vi "GeoData.vi"() -> ()   [LabVIEW 2017] (continued)
H1\n27320\t37157\tReidsville\tNC\tRockingham County\tH1\n27375\t37157\tWentworth\tNC\tRockingham County\tH1\n27357\t37157\tStokesdale\tNC\tRockingham County\tH1\n27358\t37157\tSummerfield\tNC\tRockingham County\tH1\n27214\t37157\tBrowns summit\tNC\tRockingham County\tH1\n27288\t37157\tEden\tNC\tRockingham County\tH1\n27027\t37157\tMayodan\tNC\tRockingham County\tH1\n27025\t37157\tMadison\tNC\tRockingham County\tH1\n27249\t37157\tGibsonville\tNC\tRockingham County\tH1\n27289\t37157\tEden\tNC\tRockingham County\tH1\n27311\t37157\tPelham\tNC\tRockingham County\tH1\n28147\t37159\tSalisbury\tNC\tRowan County\tH1\n28159\t37159\tSpencer\tNC\tRowan County\tH1\n28039\t37159\tEast spencer\tNC\tRowan County\tH1\n28146\t37159\tSalisbury\tNC\tRowan County\tH1\n27054\t37159\tWoodleaf\tNC\tRowan County\tH1\n28023\t37159\tChina grove\tNC\tRowan County\tH1\n28127\t37159\tNew london\tNC\tRowan County\tH1\n28072\t37159\tGranite quarry\tNC\tRowan County\tH1\n28083\t37159\tKannapolis\tNC\tRowan County\tH1\n28137\t37159\tRichfield\tNC\tRowan County\tH1\n28071\t37159\tGold hill\tNC\tRowan County\tH1\n28088\t37159\tLandis\tNC\tRowan County\tH1\n28138\t37159\tRockwell\tNC\tRowan County\tH1\n28125\t37159\tMount ulla\tNC\tRowan County\tH1\n28145\t37159\tSalisbury\tNC\tRowan County\tH1\n28625\t37159\tStatesville\tNC\tRowan County\tH1\n28036\t37159\tDavidson\tNC\tRowan County\tH1\n28081\t37159\tKannapolis\tNC\tRowan County\tH1\n28144\t37159\tSalisbury\tNC\tRowan County\tH1\n28041\t37159\tFaith\tNC\tRowan County\tH1\n27013\t37159\tCleveland\tNC\tRowan County\tH1\n28115\t37159\tMooresville\tNC\tRowan County\tH1\n28167\t37161\tUnion mills\tNC\tRutherford County\tH1\n28752\t37161\tMarion\tNC\tRutherford County\tH1\n28024\t37161\tCliffside\tNC\tRutherford County\tH1\n28139\t37161\tRutherfordton\tNC\tRutherford County\tH1\n28756\t37161\tMill spring\tNC\tRutherford County\tH1\n28076\t37161\tHenrietta\tNC\tRutherford County\tH1\n28019\t37161\tCaroleen\tNC\tRutherford County\tH1\n28746\t37161\tLake lure\tNC\tRutherford County\tH1\n28018\t37161\tBostic\tNC\tRutherford County\tH1\n28043\t37161\tForest city\tNC\tRutherford County\tH1\n28150\t37161\tShelby\tNC\tRutherford County\tH1\n28020\t37161\tCasar\tNC\tRutherford County\tH1\n28711\t37161\tBlack mountain\tNC\tRutherford County\tH1\n28160\t37161\tSpindale\tNC\tRutherford County\tH1\n28074\t37161\tHarris\tNC\tRutherford County\tH1\n28040\t37161\tEllenboro\tNC\tRutherford County\tH1\n28114\t37161\tMooresboro\tNC\tRutherford County\tH1\n28720\t37161\tChimney rock\tNC\tRutherford County\tH1\n28334\t37163\tDunn\tNC\tSampson County\tH1\n28458\t37163\tRose hill\tNC\tSampson County\tH1\n28393\t37163\tTurkey\tNC\tSampson County\tH1\n28328\t37163\tClinton\tNC\tSampson County\tH1\n28365\t37163\tMount olive\tNC\tSampson County\tH1\n28444\t37163\tHarrells\tNC\tSampson County\tH1\n28329\t37163\tClinton\tNC\tSampson County\tH1\n28366\t37163\tNewton grove\tNC\tSampson County\tH1\n28385\t37163\tSalemburg\tNC\tSampson County\tH1\n28341\t37163\tFaison\tNC\tSampson County\tH1\n28344\t37163\tGodwin\tNC\tSampson County\tH1\n28453\t37163\tMagnolia\tNC\tSampson County\tH1\n28382\t37163\tRoseboro\tNC\tSampson County\tH1\n28391\t37163\tStedman\tNC\tSampson County\tH1\n28398\t37163\tWarsaw\tNC\tSampson County\tH1\n28447\t37163\tIvanhoe\tNC\tSampson County\tH1\n28318\t37163\tAutryville\tNC\tSampson County\tH1\n28478\t37163\tWillard\tNC\tSampson County\tH1\n28421\t37163\tAtkinson\tNC\tSampson County\tH1\n28441\t37163\tGarland\tNC\tSampson County\tH1\n28466\t37163\tWallace\tNC\tSampson County\tH1\n28352\t37165\tLaurinburg\tNC\tScotland County\tH1\n28364\t37165\tMaxton\tNC\tScotland County\tH1\n28396\t37165\tWagram\tNC\tScotland County\tH1\n28363\t37165\tMarston\tNC\tScotland County\tH1\n28351\t37165\tLaurel hill\tNC\tScotland County\tH1\n28343\t37165\tGibson\tNC\tScotland County\tH1\n28345\t37165\tHamlet\tNC\tScotland County\tH1\n28353\t37165\tLaurinburg\tNC\tScotland County\tH1\n28009\t37167\tBadin\tNC\tStanly County\tH1\n28002\t37167\tAlbemarle\tNC\tStanly County\tH1\n28127\t37167\tNew london\tNC\tStanly County\tH1\n28001\t37167\tAlbemarle\tNC\tStanly County\tH1\n28097\t37167\tLocust\tNC\tStanly County\tH1\n28129\t37167\tOakboro\tNC\tStanly County\tH1\n28163\t37167\tStanfield\tNC\tStanly County\tH1\n28137\t37167\tRichfield\tNC\tStanly County\tH1\n28109\t37167\tMisenheimer\tNC\tStanly County\tH1\n28071\t37167\tGold hill\tNC\tStanly County\tH1\n28107\t37167\tMidland\tNC\tStanly County\tH1\n28128\t37167\tNorwood\tNC\tStanly County\tH1\n28124\t37167\tMount pleasant\tNC\tStanly County\tH1\n27009\t37169\tBelews creek\tNC\tStokes County\tH1\n27046\t37169\tSandy ridge\tNC\tStokes County\tH1\n27021\t37169\tKing\tNC\tStokes County\tH1\n27043\t37169\tPinnacle\tNC\tStokes County\tH1\n27045\t37169\tRural hall\tNC\tStokes County\tH1\n27022\t37169\tLawsonville\tNC\tStokes County\tH1\n27042\t37169\tPine hall\tNC\tStokes County\tH1\n27041\t37169\tPilot mountain\tNC\tStokes County\tH1\n27019\t37169\tGermanton\tNC\tStokes County\tH1\n27053\t37169\tWestfield\tNC\tStokes County\tH1\n27052\t37169\tWalnut cove\tNC\tStokes County\tH1\n27357\t37169\tStokesdale\tNC\tStokes County\tH1\n27016\t37169\tDanbury\tNC\tStokes County\tH1\n27030\t37169\tMount airy\tNC\tStokes County\tH1\n27050\t37169\tTobaccoville\tNC\tStokes County\tH1\n27025\t37169\tMadison\tNC\tStokes County\tH1\n27043\t37171\tPinnacle\tNC\tSurry County\tH1\n27047\t37171\tSiloam\tNC\tSurry County\tH1\n28669\t37171\tRoaring river\tNC\tSurry County\tH1\n28676\t37171\tState road\tNC\tSurry County\tH1\n27024\t37171\tLowgap\tNC\tSurry County\tH1\n28621\t37171\tElkin\tNC\tSurry County\tH1\n27049\t37171\tToast\tNC\tSurry County\tH1\n27041\t37171\tPilot mountain\tNC\tSurry County\tH1\n27053\t37171\tWestfield\tNC\tSurry County\tH1\n28683\t37171\tThurmond\tNC\tSurry County\tH1\n27030\t37171\tMount airy\tNC\tSurry County\tH1\n27017\t37171\tDobson\tNC\tSurry County\tH1\n27007\t37171\tArarat\tNC\tSurry County\tH1\n28713\t37173\tBryson city\tNC\tSwain County\tH1\n28719\t37173\tCherokee\tNC\tSwain County\tH1\n28702\t37173\tAlmond\tNC\tSwain County\tH1\n28789\t37173\tWhittier\tNC\tSwain County\tH1\n28771\t37173\tRobbinsville\tNC\tSwain County\tH1\n28708\t37175\tBalsam grove\tNC\tTransylvania County\tH1\n28718\t37175\tCedar mountain\tNC\tTransylvania County\tH1\n28747\t37175\tLake toxaway\tNC\tTransylvania County\tH1\n28766\t37175\tPenrose\tNC\tTransylvania County\tH1\n28739\t37175\tHendersonville\tNC\tTransylvania County\tH1\n28742\t37175\tHorse shoe\tNC\tTransylvania County\tH1\n28712\t37175\tBrevard\tNC\tTransylvania County\tH1\n28768\t37175\tPisgah forest\tNC\tTransylvania County\tH1\n28772\t37175\tRosman\tNC\tTransylvania County\tH1\n28783\t37175\tTuckasegee\tNC\tTransylvania County\tH1\n28774\t37175\tSapphire\tNC\tTransylvania County\tH1\n28759\t37175\tMills river\tNC\tTransylvania County\tH1\n27826\t37177\tFairfield\tNC\tTyrrell County\tH1\n27925\t37177\tColumbia\tNC\tTyrrell County\tH1\n27928\t37177\tCreswell\tNC\tTyrrell County\tH1\n28108\t37179\tMineral springs\tNC\tUnion County\tH1\n28135\t37179\tPolkton\tNC\tUnion County\tH1\n28133\t37179\tPeachland\tNC\tUnion County\tH1\n28227\t37179\tCharlotte\tNC\tUnion County\tH1\n28103\t37179\tMarshville\tNC\tUnion County\tH1\n28105\t37179\tMatthews\tNC\tUnion County\tH1\n28112\t37179\tMonroe\tNC\tUnion County\tH1\n28107\t37179\tMidland\tNC\tUnion County\tH1\n28111\t37179\tMonroe\tNC\tUnion County\tH1\n28174\t37179\tWingate\tNC\tUnion County\tH1\n28079\t37179\tIndian trail\tNC\tUnion County\tH1\n28173\t37179\tWaxhaw\tNC\tUnion County\tH1\n28104\t37179\tMatthews\tNC\tUnion County\tH1\n28110\t37179\tMonroe\tNC\tUnion County\tH1\n27537\t37181\tHenderson\tNC\tVance County\tH1\n27553\t37181\tManson\tNC\tVance County\tH1\n27565\t37181\tOxford\tNC\tVance County\tH1\n27556\t37181\tMiddleburg\tNC\tVance County\tH1\n27507\t37181\tBullock\tNC\tVance County\tH1\n27536\t37181\tHenderson\tNC\tVance County\tH1\n27563\t37181\tNorlina\tNC\tVance County\tH1\n27544\t37181\tKittrell\tNC\tVance County\tH1\n27584\t37181\tTownsville\tNC\tVance County\tH1\n27512\t37183\tCary\tNC\tWake County\tH1\n27587\t37183\tWake forest\tNC\tWake County\tH1\n27610\t37183\tRaleigh\tNC\tWake County\tH1\n27614\t37183\tRaleigh\tNC\tWake County\tH1\n27640\t37183\tRaleigh\tNC\tWake County\tH1\n27502\t37183\tApex\tNC\tWake County\tH1\n27519\t37183\tCary\tNC\tWake County\tH1\n27526\t37183\tFuquay varina\tNC\tWake County\tH1\n27562\t37183\tNew hill\tNC\tWake County\tH1\n27619\t37183\tRaleigh\tNC\tWake County\tH1\n27699\t37183\tRaleigh\tNC\tWake County\tH1\n27690\t37183\tRaleigh\tNC\tWake County\tH1\n27661\t37183\tRaleigh\tNC\tWake County\tH1\n27501\t37183\tAngier\tNC\tWake County\tH1\n27604\t37183\tRaleigh\tNC\tWake County\tH1\n27596\t37183\tYoungsville\tNC\tWake County\tH1\n27713\t37183\tDurham\tNC\tWake County\tH1\n27628\t37183\tRaleigh\tNC\tWake County\tH1\n27520\t37183\tClayton\tNC\tWake County\tH1\n27518\t37183\tCary\tNC\tWake County\tH1\n27545\t37183\tKnightdale\tNC\tWake County\tH1\n27560\t37183\tMorrisville\tNC\tWake County\tH1\n27592\t37183\tWillow spring\tNC\tWake County\tH1\n27609\t37183\tRaleigh\tNC\tWake County\tH1\n27615\t37183\tRaleigh\tNC\tWake County\tH1\n27622\t37183\tRaleigh\tNC\tWake County\tH1\n27629\t37183\tRaleigh\tNC\tWake County\tH1\n27675\t37183\tRaleigh\tNC\tWake County\tH1\n27611\t37183\tRaleigh\tNC\tWake County\tH1\n27513\t37183\tCary\tNC\tWake County\tH1\n27522\t37183\tCreedmoor\tNC\tWake County\tH1\n27529\t37183\tGarner\tNC\tWake County\tH1\n27656\t37183\tRaleigh\tNC\tWake County\tH1\n27511\t37183\tCary\tNC\tWake County\tH1\n27523\t37183\tApex\tNC\tWake County\tH1\n27591\t37183\tWendell\tNC\tWake County\tH1\n27603\t37183\tRaleigh\tNC\tWake County\tH1\n27605\t37183\tRaleigh\tNC\tWake County\tH1\n27607\t37183\tRaleigh\tNC\tWake County\tH1\n27608\t37183\tRaleigh\tNC\tWake County\tH1\n27613\t37183\tRaleigh\tNC\tWake County\tH1\n27616\t37183\tRaleigh\tNC\tWake County\tH1\n27588\t37183\tWake forest\tNC\tWake County\tH1\n27636\t37183\tRaleigh\tNC\tWake County\tH1\n27697\t37183\tRaleigh\tNC\tWake County\tH1\n27602\t37183\tRaleigh\tNC\tWake County\tH1\n27601\t37183\tRaleigh\tNC\tWake County\tH1\n27606\t37183\tRaleigh\tNC\tWake County\tH1\n27612\t37183\tRaleigh\tNC\tWake County\tH1\n27617\t37183\tRaleigh\tNC\tWake County\tH1\n27703\t37183\tDurham\tNC\tWake County\tH1\n27571\t37183\tRolesville\tNC\tWake County\tH1\n27620\t37183\tRaleigh\tNC\tWake County\tH1\n27623\t37183\tRaleigh\tNC\tWake County\tH1\n27540\t37183\tHolly springs\tNC\tWake County\tH1\n27539\t37183\tApex\tNC\tWake County\tH1\n27597\t37183\tZebulon\tNC\tWake County\tH1\n27627\t37183\tRaleigh\tNC\tWake County\tH1\n27624\t37183\tRaleigh\tNC\tWake County\tH1\n27658\t37183\tRaleigh\tNC\tWake County\tH1\n27676\t37183\tRaleigh\tNC\tWake County\tH1\n27537\t37185\tHenderson\tNC\tWarren County\tH1\n27551\t37185\tMacon\tNC\tWarren County\tH1\n27553\t37185\tManson\tNC\tWarren County\tH1\n27850\t37185\tLittleton\tNC\tWarren County\tH1\n27589\t37185\tWarrenton\tNC\tWarren County\tH1\n27844\t37185\tHollister\tNC\tWarren County\tH1\n27586\t37185\tVaughan\tNC\tWarren County\tH1\n27563\t37185\tNorlina\tNC\tWarren County\tH1\n27594\t37185\tWise\tNC\tWarren County\tH1\n27570\t37185\tRidgeway\tNC\tWarren County\tH1\n27842\t37185\tHenrico\tNC\tWarren County\tH1\n27860\t37187\tPantego\tNC\tWashington County\tH1\n27962\t37187\tPlymouth\tNC\tWashington County\tH1\n27970\t37187\tRoper\tNC\tWashington County\tH1\n27928\t37187\tCreswell\tNC\tWashington County\tH1\n27865\t37187\tPinetown\tNC\tWashington County\tH1\n28622\t37189\tElk park\tNC\tWatauga County\tH1\n28604\t37189\tBanner elk\tNC\tWatauga County\tH1\n28645\t37189\tLenoir\tNC\tWatauga County\tH1\n28608\t37189\tBoone\tNC\tWatauga County\tH1\n28698\t37189\tZionville\tNC\tWatauga County\tH1\n28607\t37189\tBoone\tNC\tWatauga County\tH1\n28605\t37189\tBlowing rock\tNC\tWatauga County\tH1\n28692\t37189\tVilas\tNC\tWatauga County\tH1\n28618\t37189\tDeep gap\tNC\tWatauga County\tH1\n28684\t37189\tTodd\tNC\tWatauga County\tH1\n28679\t37189\tSugar grove\tNC\tWatauga County\tH1\n27542\t37191\tKenly\tNC\tWayne County\tH1\n27524\t37191\tFour oaks\tNC\tWayne County\tH1\n27863\t37191\tPikeville\tNC\tWayne County\tH1\n28333\t37191\tDudley\tNC\tWayne County\tH1\n28365\t37191\tMount olive\tNC\tWayne County\tH1\n27533\t37191\tGoldsboro\tNC\tWayne County\tH1\n27569\t37191\tPrinceton\tNC\tWayne County\tH1\n27531\t37191\tGoldsboro\tNC\tWayne County\tH1\n27830\t37191\tFremont\tNC\tWayne County\tH1\n28578\t37191\tSeven springs\tNC\tWayne County\tH1\n27532\t37191\tGoldsboro\tNC\tWayne County\tH1\n27534\t37191\tGoldsboro\tNC\tWayne County\tH1\n27851\t37191\tLucama\tNC\tWayne County\tH1\n27530\t37191\tGoldsboro\tNC\tWayne County\tH1\n27883\t37191\tStantonsburg\tNC\tWayne County\tH1\n28551\t37191\tLa grange\tNC\tWayne County\tH1\n28635\t37193\tHays\tNC\tWilkes County\tH1\n28651\t37193\tMillers creek\tNC\tWilkes County\tH1\n28670\t37193\tRonda\tNC\tWilkes County\tH1\n28624\t37193\tFerguson\tNC\tWilkes County\tH1\n28645\t37193\tLenoir\tNC\tWilkes County\tH1\n28644\t37193\tLaurel springs\tNC\tWilkes County\tH1\n28669\t37193\tRoaring river\tNC\tWilkes County\tH1\n28676\t37193\tState road\tNC\tWilkes County\tH1\n28621\t37193\tElkin\tNC\tWilkes County\tH1\n28659\t37193\tNorth wilkesboro\tNC\tWilkes County\tH1\n28654\t37193\tMoravian falls\tNC\tWilkes County\tH1\n28642\t37193\tJonesville\tNC\tWilkes County\tH1\n28685\t37193\tTraphill\tNC\tWilkes County\tH1\n28683\t37193\tThurmond\tNC\tWilkes County\tH1\n28618\t37193\tDeep gap\tNC\tWilkes County\tH1\n28665\t37193\tPurlear\tNC\tWilkes County\tH1\n28649\t37193\tMc grady\tNC\tWilkes County\tH1\n28606\t37193\tBoomer\tNC\tWilkes County\tH1\n28694\t37193\tWest jefferson\tNC\tWilkes County\tH1\n27020\t37193\tHamptonville\tNC\tWilkes County\tH1\n28697\t37193\tWilkesboro\tNC\tWilkes County\tH1\n28689\t37193\tUnion grove\tNC\tWilkes County\tH1\n28656\t37193\tNorth wilkesboro\tNC\tWilkes County\tH1\n27542\t37195\tKenly\tNC\tWilson County\tH1\n27894\t37195\tWilson\tNC\tWilson County\tH1\n27803\t37195\tRocky mount\tNC\tWilson County\tH1\n27807\t37195\tBailey\tNC\tWilson County\tH1\n27852\t37195\tMacclesfield\tNC\tWilson County\tH1\n27822\t37195\tElm city\tNC\tWilson County\tH1\n27880\t37195\tSims\tNC\tWilson County\tH1\n27893\t37195\tWilson\tNC\tWilson County\tH1\n27829\t37195\tFountain\tNC\tWilson County\tH1\n27888\t37195\tWalstonburg\tNC\tWilson County\tH1\n27830\t37195\tFremont\tNC\tWilson County\tH1\n27895\t37195\tWilson\tNC\tWilson County\tH1\n27873\t37195\tSaratoga\tNC\tWilson County\tH1\n27896\t37195\tWilson\tNC\tWilson County\tH1\n27813\t37195\tBlack creek\tNC\tWilson County\tH1\n27851\t37195\tLucama\tNC\tWilson County\tH1\n27557\t37195\tMiddlesex\tNC\tWilson County\tH1\n27883\t37195\tStantonsburg\tNC\tWilson County\tH1\n27011\t37197\tBoonville\tNC\tYadkin County\tH1\n28634\t37197\tHarmony\tNC\tYadkin County\tH1\n27018\t37197\tEast bend\tNC\tYadkin County\tH1\n28642\t37197\tJonesville\tNC\tYadkin County\tH1\n27020\t37197\tHamptonville\tNC\tYadkin County\tH1\n27055\t37197\tYadkinville\tNC\tYadkin County\tH1\n28689\t37197\tUnion grove\tNC\tYadkin County\tH1\n28714\t37199\tBurnsville\tNC\tYancey County\tH1\n28777\t37199\tSpruce pine\tNC\tYancey County\tH1\n28755\t37199\tMicaville\tNC\tYancey County\tH1\n28740\t37199\tGreen mountain\tNC\tYancey County\tH1\n28754\t37199\tMars hill\tNC\tYancey County\tH1\n28705\t37199\tBakersville\tNC\tYancey County\tH1\n58639\t38001\tHettinger\tND\tAdams County\tH1\n58562\t38001\tNew leipzig\tND\tAdams County\tH1\n58649\t38001\tReeder\tND\tAdams County\tH1\n58646\t38001\tMott\tND\tAdams County\tH1\n58650\t38001\tRegent\tND\tAdams County\tH1\n58479\t38003\tRogers\tND\tBarnes County\tH1\n58492\t38003\tWimbledon\tND\tBarnes County\tH1\n58466\t38003\tMarion\tND\tBarnes County\tH1\n58065\t38003\tPillsbury\tND\tBarnes County\tH1\n58072\t38003\tValley city\tND\tBarnes County\tH1\n58062\t38003\tNome\tND\tBarnes County\tH1\n58481\t38003\tSpiritwood\tND\tBarnes County\tH1\n58031\t38003\tFingal\tND\tBarnes County\tH1\n58056\t38003\tLuverne\tND\tBarnes County\tH1\n58497\t38003\tYpsilanti\tND\tBarnes County\tH1\n58064\t38003\tPage\tND\tBarnes County\tH1\n58049\t38003\tKathryn\tND\tBarnes County\tH1\n58027\t38003\tEnderlin\tND\tBarnes County\tH1\n58071\t38003\tTower city\tND\tBarnes County\tH1\n58063\t38003\tOriska\tND\tBarnes County\tH1\n58461\t38003\tLitchville\tND\tBarnes County\tH1\n58480\t38003\tSanborn\tND\tBarnes County\tH1\n58046\t38003\tHope\tND\tBarnes County\tH1\n58429\t38003\tDazey\tND\tBarnes County\tH1\n58374\t38005\tSheyenne\tND\tBenson County\tH1\n58348\t38005\tMaddock\tND\tBenson County\tH1\n58381\t38005\tWarwick\tND\tBenson County\tH1\n58357\t38005\tOberon\tND\tBenson County\tH1\n58335\t38005\tFort totten\tND\tBenson County\tH1\n58301\t38005\tDevils lake\tND\tBenson County\tH1\n58332\t38005\tEsmond\tND\tBenson County\tH1\n58370\t38005\tSaint michael\tND\tBenson County\tH1\n58368\t38005\tRugby\tND\tBenson County\tH1\n58386\t38005\tYork\tND\tBenson County\tH1\n58343\t38005\tKnox\tND\tBenson County\tH1\n58325\t38005\tChurchs ferry\tND\tBenson County\tH1\n58380\t38005\tTolna\tND\tBenson County\tH1\n58341\t38005\tHarvey\tND\tBenson County\tH1\n58385\t38005\tWolford\tND\tBenson County\tH1\n58346\t38005\tLeeds\tND\tBenson County\tH1\n58351\t38005\tMinnewaukan\tND\tBenson County\tH1\n58379\t38005\tTokio\tND\tBenson County\tH1\n58622\t38007\tBelfield\tND\tBillings County\tH1\n58620\t38007\tAmidon\tND\tBillings County\tH1\n58645\t38007\tMedora\tND\tBillings County\tH1\n58640\t38007\tKilldeer\tND\tBillings County\tH1\n58627\t38007\tFairfield\tND\tBillings County\tH1\n58634\t38007\tGrassy butte\tND\tBillings County\tH1\n58642\t38007\tManning\tND\tBillings County\tH1\n58750\t38009\tLansford\tND\tBottineau County\tH1\n58740\t38009\tGlenburn\tND\tBottineau County\tH1\n58711\t38009\tAntler\tND\tBottineau County\tH1\n58762\t38009\tNewburg\tND\tBottineau County\tH1\n58384\t38009\tWillow city\tND\tBottineau County\tH1\n58760\t38009\tMaxbass\tND\tBottineau County\tH1\n58318\t38009\tBottineau\tND\tBottineau County\tH1\n58782\t38009\tSherwood\tND\tBottineau County\tH1\n58783\t38009\tSouris\tND\tBottineau County\tH1\n58789\t38009\tUpham\tND\tBottineau County\tH1\n58793\t38009\tWesthope\tND\tBottineau County\tH1\n58329\t38009\tDunseith\tND\tBottineau County\tH1\n58761\t38009\tMohall\tND\tBottineau County\tH1\n58748\t38009\tKramer\tND\tBottineau County\tH1\n58643\t38011\tMarmarth\tND\tBowman County\tH1\n58651\t38011\tRhame\tND\tBowman County\tH1\n58653\t38011\tScranton\tND\tBowman County\tH1\n58623\t38011\tBowman\tND\tBowman County\tH1\n58649\t38011\tReeder\tND\tBowman County\tH1\n58737\t38013\tFlaxton\tND\tBurke County\tH1\n58784\t38013\tStanley\tND\tBurke County\tH1\n58727\t38013\tColumbus\tND\tBurke County\tH1\n58772\t38013\tPortal\tND\tBurke County\tH1\n58755\t38013\tMcgregor\tND\tBurke County\tH1\n58721\t38013\tBowbells\tND\tBurke County\tH1\n58773\t38013\tPowers lake\tND\tBurke County\tH1\n58752\t38013\tLignite\tND\tBurke County\tH1\n58746\t38013\tKenmare\tND\tBurke County\tH1\n58504\t38015\tBismarck\tND\tBurleigh County\tH1\n58521\t38015\tBaldwin\tND\tBurleigh County\tH1\n58505\t38015\tBismarck\tND\tBurleigh County\tH1\n58501\t38015\tBismarck\tND\tBurleigh County\tH1\n58524\t38015\tBraddock\tND\tBurleigh County\tH1\n58572\t38015\tSterling\tND\tBurleigh County\tH1\n58579\t38015\tWilton\tND\tBurleigh County\tH1\n58502\t38015\tBismarck\tND\tBurleigh County\tH1\n58494\t38015\tWing\tND\tBurleigh County\tH1\n58532\t38015\tDriscoll\tND\tBurleigh County\tH1\n58477\t38015\tRegan\tND\tBurleigh County\tH1\n58560\t38015\tMoffit\tND\tBurleigh County\tH1\n58503\t38015\tBismarck\tND\tBurleigh County\tH1\n58506\t38015\tBismarck\tND\tBurleigh County\tH1\n58558\t38015\tMenoken\tND\tBurleigh County\tH1\n58507\t38015\tBismarck\tND\tBurleigh County\tH1\n58103\t38017\tFargo\tND\tCass County\tH1\n58006\t38017\tArthur\tND\tCass County\tH1\n58038\t38017\tGrandin\tND\tCass County\tH1\n58042\t38017\tHarwood\tND\tCass County\tH1\n58126\t38017\tFargo\tND\tCass County\tH1\n58047\t38017\tHorace\tND\tCass County\tH1\n58012\t38017\tCasselton\tND\tCass County\tH1\n58015\t38017\tChristine\tND\tCass County\tH1\n58104\t38017\tFargo\tND\tCass County\tH1\n58035\t38017\tGalesburg\tND\tCass County\tH1\n58105\t38017\tFargo\tND\tCass County\tH1\n58079\t38017\tWheatland\tND\tCass County\tH1\n58106\t38017\tFargo\tND\tCass County\tH1\n58002\t38017\tAbsaraka\tND\tCass County\tH1\n58031\t38017\tFingal\tND\tCass County\tH1\n58064\t38017\tPage\tND\tCass County\tH1\n58108\t38017\tFargo\tND\tCass County\tH1\n58125\t38017\tFargo\tND\tCass County\tH1\n58124\t38017\tFargo\tND\tCass County\tH1\n58027\t38017\tEnderlin\tND\tCass County\tH1\n58107\t38017\tFargo\tND\tCass County\tH1\n58048\t38017\tHunter\tND\tCass County\tH1\n58021\t38017\tDavenport\tND\tCass County\tH1\n58071\t38017\tTower city\tND\tCass County\tH1\n58004\t38017\tAmenia\tND\tCass County\tH1\n58109\t38017\tFargo\tND\tCass County\tH1\n58121\t38017\tFargo\tND\tCass County\tH1\n58078\t38017\tWest fargo\tND\tCass County\tH1\n58052\t38017\tLeonard\tND\tCass County\tH1\n58011\t38017\tBuffalo\tND\tCass County\tH1\n58029\t38017\tErie\tND\tCass County\tH1\n58051\t38017\tKindred\tND\tCass County\tH1\n58046\t38017\tHope\tND\tCass County\tH1\n58007\t38017\tAyr\tND\tCass County\tH1\n58036\t38017\tGardner\tND\tCass County\tH1\n58122\t38017\tFargo\tND\tCass County\tH1\n58102\t38017\tFargo\tND\tCass County\tH1\n58059\t38017\tMapleton\tND\tCass County\tH1\n58005\t38017\tArgusville\tND\tCass County\tH1\n58239\t38019\tHannah\tND\tCavalier County\tH1\n58330\t38019\tEdmore\tND\tCavalier County\tH1\n58338\t38019\tHampden\tND\tCavalier County\tH1\n58282\t38019\tWalhalla\tND\tCavalier County\tH1\n58377\t38019\tStarkweather\tND\tCavalier County\tH1\n58227\t38019\tEdinburg\tND\tCavalier County\tH1\n58352\t38019\tMunich\tND\tCavalier County\tH1\n58281\t38019\tWales\tND\tCavalier County\tH1\n58255\t38019\tMaida\tND\tCavalier County\tH1\n58269\t38019\tOsnabrock\tND\tCavalier County\tH1\n58260\t38019\tMilton\tND\tCavalier County\tH1\n58249\t38019\tLangdon\tND\tCavalier County\tH1\n58229\t38019\tFairdale\tND\tCavalier County\tH1\n58372\t38019\tSarles\tND\tCavalier County\tH1\n58311\t38019\tAlsen\tND\tCavalier County\tH1\n58262\t38019\tMountain\tND\tCavalier County\tH1\n58355\t38019\tNekoma\tND\tCavalier County\tH1\n58323\t38019\tCalvin\tND\tCavalier County\tH1\n58040\t38021\tGwinner\tND\tDickey County\tH1\n58439\t38021\tForbes\tND\tDickey County\tH1\n58456\t38021\tKulm\tND\tDickey County\tH1\n58436\t38021\tEllendale\tND\tDickey County\tH1\n58474\t38021\tOakes\tND\tDickey County\tH1\n58458\t38021\tLamoure\tND\tDickey County\tH1\n58441\t38021\tFullerton\tND\tDickey County\tH1\n58413\t38021\tAshley\tND\tDickey County\tH1\n58433\t38021\tEdgeley\tND\tDickey County\tH1\n58415\t38021\tBerlin\tND\tDickey County\tH1\n58845\t38023\tGrenora\tND\tDivide County\tH1\n58833\t38023\tAmbrose\tND\tDivide County\tH1\n58856\t38023\tZahl\tND\tDivide County\tH1\n58765\t38023\tNoonan\tND\tDivide County\tH1\n58755\t38023\tMcgregor\tND\tDivide County\tH1\n58830\t38023\tAlamo\tND\tDivide County\tH1\n58795\t38023\tWildrose\tND\tDivide County\tH1\n58730\t38023\tCrosby\tND\tDivide County\tH1\n58844\t38023\tFortuna\tND\tDivide County\tH1\n58601\t38025\tDickinson\tND\tDunn County\tH1\n58638\t38025\tHebron\tND\tDunn County\tH1\n58625\t38025\tDodge\tND\tDunn County\tH1\n58757\t38025\tMandaree\tND\tDunn County\tH1\n58636\t38025\tHalliday\tND\tDunn County\tH1\n58656\t38025\tTaylor\tND\tDunn County\tH1\n58626\t38025\tDunn center\tND\tDunn County\tH1\n58622\t38025\tBelfield\tND\tDunn County\tH1\n58644\t38025\tMarshall\tND\tDunn County\tH1\n58652\t38025\tRichardton\tND\tDunn County\tH1\n58640\t38025\tKilldeer\tND\tDunn County\tH1\n58854\t38025\tWatford city\tND\tDunn County\tH1\n58630\t38025\tGladstone\tND\tDunn County\tH1\n58642\t38025\tManning\tND\tDunn County\tH1\n58374\t38027\tSheyenne\tND\tEddy County\tH1\n58421\t38027\tCarrington\tND\tEddy County\tH1\n58381\t38027\tWarwick\tND\tEddy County\tH1\n58356\t38027\tNew rockford\tND\tEddy County\tH1\n58445\t38027\tGrace city\tND\tEddy County\tH1\n58380\t38027\tTolna\tND\tEddy County\tH1\n58464\t38027\tMchenry\tND\tEddy County\tH1\n58504\t38029\tBismarck\tND\tEmmons County\tH1\n58552\t38029\tLinton\tND\tEmmons County\tH1\n58524\t38029\tBraddock\tND\tEmmons County\tH1\n58544\t38029\tHazelton\tND\tEmmons County\tH1\n58549\t38029\tKintyre\tND\tEmmons County\tH1\n58581\t38029\tZeeland\tND\tEmmons County\tH1\n58495\t38029\tWishek\tND\tEmmons County\tH1\n58542\t38029\tHague\tND\tEmmons County\tH1\n58560\t38029\tMoffit\tND\tEmmons County\tH1\n58573\t38029\tStrasburg\tND\tEmmons County\tH1\n58443\t38031\tGlenfield\tND\tFoster County\tH1\n58421\t38031\tCarrington\tND\tFoster County\tH1\n58356\t38031\tNew rockford\tND\tFoster County\tH1\n58484\t38031\tSutton\tND\tFoster County\tH1\n58445\t38031\tGrace city\tND\tFoster County\tH1\n58464\t38031\tMchenry\tND\tFoster County\tH1\n58455\t38031\tKensal\tND\tFoster County\tH1\n58632\t38033\tGolva\tND\tGolden Valley County\tH1\n58645\t38033\tMedora\tND\tGolden Valley County\tH1\n58654\t38033\tSentinel butte\tND\tGolden Valley County\tH1\n58621\t38033\tBeach\tND\tGolden Valley County\tH1\n58261\t38035\tMinto\tND\tGrand Forks County\tH1\n58212\t38035\tAneta\tND\tGrand Forks County\tH1\n58228\t38035\tEmerado\tND\tGrand Forks County\tH1\n58278\t38035\tThompson\tND\tGrand Forks County\tH1\n58207\t38035\tGrand forks\tND\tGrand Forks County\tH1\n58256\t38035\tManvel\tND\tGrand Forks County\tH1\n58258\t38035\tMekinock\tND\tGrand Forks County\tH1\n58206\t38035\tGrand forks\tND\tGrand Forks County\tH1\n58203\t38035\tGrand forks\tND\tGrand Forks County\tH1\n58202\t38035\tGrand forks\tND\tGrand Forks County\tH1\n58231\t38035\tFordville\tND\tGrand Forks County\tH1\n58275\t38035\tReynolds\tND\tGrand Forks County\tH1\n58267\t38035\tNorthwood\tND\tGrand Forks County\tH1\n58205\t38035\tGrand forks afb\tND\tGrand Forks County\tH1\n58240\t38035\tHatton\tND\tGrand Forks County\tH1\n58266\t38035\tNiagara\tND\tGrand Forks County\tH1\n58201\t38035\tGrand forks\tND\tGrand Forks County\tH1\n58251\t38035\tLarimore\tND\tGrand Forks County\tH1\n58214\t38035\tArvilla\tND\tGrand Forks County\tH1\n58244\t38035\tInkster\tND\tGrand Forks County\tH1\n58204\t38035\tGrand forks afb\tND\tGrand Forks County\tH1\n58233\t38035\tForest river\tND\tGrand Forks County\tH1\n58208\t38035\tGrand forks\tND\tGrand Forks County\tH1\n58235\t38035\tGilby\tND\tGrand Forks County\tH1\n58638\t38037\tHebron\tND\tGrant County\tH1\n58569\t38037\tShields\tND\tGrant County\tH1\n58535\t38037\tFlasher\tND\tGrant County\tH1\n58520\t38037\tAlmont\tND\tGrant County\tH1\n58563\t38037\tNew salem\tND\tGrant County\tH1\n58562\t38037\tNew leipzig\tND\tGrant County\tH1\n58564\t38037\tRaleigh\tND\tGrant County\tH1\n58529\t38037\tCarson\tND\tGrant County\tH1\n58631\t38037\tGlen ullin\tND\tGrant County\tH1\n58533\t38037\tElgin\tND\tGrant County\tH1\n58212\t38039\tAneta\tND\tGriggs County\tH1\n58492\t38039\tWimbledon\tND\tGriggs County\tH1\n58416\t38039\tBinford\tND\tGriggs County\tH1\n58484\t38039\tSutton\tND\tGriggs County\tH1\n58056\t38039\tLuverne\tND\tGriggs County\tH1\n58448\t38039\tHannaford\tND\tGriggs County\tH1\n58464\t38039\tMchenry\tND\tGriggs County\tH1\n58425\t38039\tCooperstown\tND\tGriggs County\tH1\n58429\t38039\tDazey\tND\tGriggs County\tH1\n58452\t38039\tJessie\tND\tGriggs County\tH1\n58647\t38041\tNew england\tND\tHettinger County\tH1\n58562\t38041\tNew leipzig\tND\tHettinger County\tH1\n58646\t38041\tMott\tND\tHettinger County\tH1\n58650\t38041\tRegent\tND\tHettinger County\tH1\n58488\t38043\tTuttle\tND\tKidder County\tH1\n58524\t38043\tBraddock\tND\tKidder County\tH1\n58467\t38043\tMedina\tND\tKidder County\tH1\n58428\t38043\tDawson\tND\tKidder County\tH1\n58482\t38043\tSteele\tND\tKidder County\tH1\n58418\t38043\tBowdon\tND\tKidder County\tH1\n58549\t38043\tKintyre\tND\tKidder County\tH1\n58423\t38043\tChaseley\tND\tKidder County\tH1\n58483\t38043\tStreeter\tND\tKidder County\tH1\n58475\t38043\tPettibone\tND\tKidder County\tH1\n58532\t38043\tDriscoll\tND\tKidder County\tH1\n58496\t38043\tWoodworth\tND\tKidder County\tH1\n58478\t38043\tRobinson\tND\tKidder County\tH1\n58487\t38043\tTappen\tND\tKidder County\tH1\n58561\t38043\tNapoleon\tND\tKidder County\tH1\n58472\t38045\tMontpelier\tND\tLaMoure County\tH1\n58456\t38045\tKulm\tND\tLaMoure County\tH1\n58474\t38045\tOakes\tND\tLaMoure County\tH1\n58458\t38045\tLamoure\tND\tLaMoure County\tH1\n58466\t38045\tMarion\tND\tLaMoure County\tH1\n58490\t38045\tVerona\tND\tLaMoure County\tH1\n58033\t38045\tFort ransom\tND\tLaMoure County\tH1\n58431\t38045\tDickey\tND\tLaMoure County\tH1\n58049\t38045\tKathryn\tND\tLaMoure County\tH1\n58433\t38045\tEdgeley\tND\tLaMoure County\tH1\n58454\t38045\tJud\tND\tLaMoure County\tH1\n58461\t38045\tLitchville\tND\tLaMoure County\tH1\n58415\t38045\tBerlin\tND\tLaMoure County\tH1\n58442\t38045\tGackle\tND\tLaMoure County\tH1\n58440\t38047\tFredonia\tND\tLogan County\tH1\n58549\t38047\tKintyre\tND\tLogan County\tH1\n58483\t38047\tStreeter\tND\tLogan County\tH1\n58454\t38047\tJud\tND\tLogan County\tH1\n58460\t38047\tLehr\tND\tLogan County\tH1\n58495\t38047\tWishek\tND\tLogan County\tH1\n58561\t38047\tNapoleon\tND\tLogan County\tH1\n58442\t38047\tGackle\tND\tLogan County\tH1\n58768\t38049\tNorwich\tND\tMcHenry County\tH1\n58731\t38049\tDeering\tND\tMcHenry County\tH1\n58713\t38049\tBantry\tND\tMcHenry County\tH1\n58736\t38049\tDrake\tND\tMcHenry County\tH1\n58740\t38049\tGlenburn\tND\tMcHenry County\tH1\n58792\t38049\tVoltaire\tND\tMcHenry County\tH1\n58762\t38049\tNewburg\tND\tMcHenry County\tH1\n58384\t38049\tWillow city\tND\tMcHenry County\tH1\n58723\t38049\tButte\tND\tMcHenry County\tH1\n58741\t38049\tGranville\tND\tMcHenry County\tH1\n58712\t38049\tBalfour\tND\tMcHenry County\tH1\n58368\t38049\tRugby\tND\tMcHenry County\tH1\n58789\t38049\tUpham\tND\tMcHenry County\tH1\n58790\t38049\tVelva\tND\tMcHenry County\tH1\n58710\t38049\tAnamoose\tND\tMcHenry County\tH1\n58758\t38049\tMartin\tND\tMcHenry County\tH1\n58788\t38049\tTowner\tND\tMcHenry County\tH1\n58748\t38049\tKramer\tND\tMcHenry County\tH1\n58778\t38049\tRuso\tND\tMcHenry County\tH1\n58744\t38049\tKarlsruhe\tND\tMcHenry County\tH1\n58440\t38051\tFredonia\tND\tMcIntosh County\tH1\n58456\t38051\tKulm\tND\tMcIntosh County\tH1\n58413\t38051\tAshley\tND\tMcIntosh County\tH1\n58581\t38051\tZeeland\tND\tMcIntosh County\tH1\n58460\t38051\tLehr\tND\tMcIntosh County\tH1\n58495\t38051\tWishek\tND\tMcIntosh County\tH1\n58757\t38053\tMandaree\tND\tMcKenzie County\tH1\n58640\t38053\tKilldeer\tND\tMcKenzie County\tH1\n58835\t38053\tArnegard\tND\tMcKenzie County\tH1\n58838\t38053\tCartwright\tND\tMcKenzie County\tH1\n58847\t38053\tKeene\tND\tMcKenzie County\tH1\n58831\t38053\tAlexander\tND\tMcKenzie County\tH1\n58763\t38053\tNew town\tND\tMcKenzie County\tH1\n58854\t38053\tWatford city\tND\tMcKenzie County\tH1\n58634\t38053\tGrassy butte\tND\tMcKenzie County\tH1\n58621\t38053\tBeach\tND\tMcKenzie County\tH1\n58779\t38055\tRyder\tND\tMcLean County\tH1\n58759\t38055\tMax\tND\tMcLean County\tH1\n58540\t38055\tGarrison\tND\tMcLean County\tH1\n58771\t38055\tPlaza\tND\tMcLean County\tH1\n58576\t38055\tUnderwood\tND\tMcLean County\tH1\n58531\t38055\tColeharbor\tND\tMcLean County\tH1\n58756\t38055\tMakoti\tND\tMcLean County\tH1\n58579\t38055\tWilton\tND\tMcLean County\tH1\n58770\t38055\tParshall\tND\tMcLean County\tH1\n58723\t38055\tButte\tND\tMcLean County\tH1\n58775\t38055\tRoseglen\tND\tMcLean County\tH1\n58716\t38055\tBenedict\tND\tMcLean County\tH1\n58559\t38055\tMercer\tND\tMcLean County\tH1\n58575\t38055\tTurtle lake\tND\tMcLean County\tH1\n58735\t38055\tDouglas\tND\tMcLean County\tH1\n58577\t38055\tWashburn\tND\tMcLean County\tH1\n58565\t38055\tRiverdale\tND\tMcLean County\tH1\n58778\t38055\tRuso\tND\tMcLean County\tH1\n58638\t38057\tHebron\tND\tMercer County\tH1\n58625\t38057\tDodge\tND\tMercer County\tH1\n58530\t38057\tCenter\tND\tMercer County\tH1\n58580\t38057\tZap\tND\tMercer County\tH1\n58541\t38057\tGolden valley\tND\tMercer County\tH1\n58523\t38057\tBeulah\tND\tMercer County\tH1\n58545\t38057\tHazen\tND\tMercer County\tH1\n58631\t38057\tGlen ullin\tND\tMercer County\tH1\n58571\t38057\tStanton\tND\tMercer County\tH1\n58638\t38059\tHebron\tND\tMorton County\tH1\n58569\t38059\tShields\tND\tMorton County\tH1\n58535\t38059\tFlasher\tND\tMorton County\tH1\n58520\t38059\tAlmont\tND\tMorton County\tH1\n58554\t38059\tMandan\tND\tMorton County\tH1\n58563\t38059\tNew salem\tND\tMorton County\tH1\n58631\t38059\tGlen ullin\tND\tMorton County\tH1\n58566\t38059\tSaint anthony\tND\tMorton County\tH1\n58570\t38059\tSolen\tND\tMorton County\tH1\n58771\t38061\tPlaza\tND\tMountrail County\tH1\n58784\t38061\tStanley\tND\tMountrail County\tH1\n58756\t38061\tMakoti\tND\tMountrail County\tH1\n58770\t38061\tParshall\tND\tMountrail County\tH1\n58718\t38061\tBerthold\tND\tMountrail County\tH1\n58734\t38061\tDonnybrook\tND\tMountrail County\tH1\n58725\t38061\tCarpio\tND\tMountrail County\tH1\n58773\t38061\tPowers lake\tND\tMountrail County\tH1\n58776\t38061\tRoss\tND\tMountrail County\tH1\n58763\t38061\tNew town\tND\tMountrail County\tH1\n58794\t38061\tWhite earth\tND\tMountrail County\tH1\n58852\t38061\tTioga\tND\tMountrail County\tH1\n58769\t38061\tPalermo\tND\tMountrail County\tH1\n58746\t38061\tKenmare\tND\tMountrail County\tH1\n58259\t38063\tMichigan\tND\tNelson County\tH1\n58327\t38063\tCrary\tND\tNelson County\tH1\n58212\t38063\tAneta\tND\tNelson County\tH1\n58321\t38063\tBrocket\tND\tNelson County\tH1\n58344\t38063\tLakota\tND\tNelson County\tH1\n58224\t38063\tDahlen\tND\tNelson County\tH1\n58266\t38063\tNiagara\tND\tNelson County\tH1\n58380\t38063\tTolna\tND\tNelson County\tH1\n58361\t38063\tPekin\tND\tNelson County\tH1\n58272\t38063\tPetersburg\tND\tNelson County\tH1\n58254\t38063\tMcville\tND\tNelson County\tH1\n58530\t38065\tCenter\tND\tOliver County\tH1\n58563\t38065\tNew salem\tND\tOliver County\tH1\n58523\t38065\tBeulah\tND\tOliver County\tH1\n58545\t38065\tHazen\tND\tOliver County\tH1\n58571\t38065\tStanton\tND\tOliver County\tH1\n58282\t38067\tWalhalla\tND\tPembina County\tH1\n58276\t38067\tSaint thomas\tND\tPembina County\tH1\n58227\t38067\tEdinburg\tND\tPembina County\tH1\n58265\t38067\tNeche\tND\tPembina County\tH1\n58238\t38067\tHamilton\tND\tPembina County\tH1\n58271\t38067\tPembina\tND\tPembina County\tH1\n58220\t38067\tCavalier\tND\tPembina County\tH1\n58243\t38067\tHoople\tND\tPembina County\tH1\n58216\t38067\tBathgate\tND\tPembina County\tH1\n58236\t38067\tGlasston\tND\tPembina County\tH1\n58225\t38067\tDrayton\tND\tPembina County\tH1\n58241\t38067\tHensel\tND\tPembina County\tH1\n58262\t38067\tMountain\tND\tPembina County\tH1\n58222\t38067\tCrystal\tND\tPembina County\tH1\n58384\t38069\tWillow city\tND\tPierce County\tH1\n58332\t38069\tEsmond\tND\tPierce County\tH1\n58368\t38069\tRugby\tND\tPierce County\tH1\n58386\t38069\tYork\tND\tPierce County\tH1\n58710\t38069\tAnamoose\tND\tPierce County\tH1\n58313\t38069\tBalta\tND\tPierce County\tH1\n58341\t38069\tHarvey\tND\tPierce County\tH1\n58758\t38069\tMartin\tND\tPierce County\tH1\n58385\t38069\tWolford\tND\tPierce County\tH1\n58346\t38069\tLeeds\tND\tPierce County\tH1\n58366\t38069\tRolette\tND\tPierce County\tH1\n58788\t38069\tTowner\tND\tPierce County\tH1\n58327\t38071\tCrary\tND\tRamsey County\tH1\n58330\t38071\tEdmore\tND\tRamsey County\tH1\n58338\t38071\tHampden\tND\tRamsey County\tH1\n58324\t38071\tCando\tND\tRamsey County\tH1\n58377\t38071\tStarkweather\tND\tRamsey County\tH1\n58381\t38071\tWarwick\tND\tRamsey County\tH1\n58301\t38071\tDevils lake\tND\tRamsey County\tH1\n58321\t38071\tBrocket\tND\tRamsey County\tH1\n58344\t38071\tLakota\tND\tRamsey County\tH1\n58362\t38071\tPenn\tND\tRamsey County\tH1\n58382\t38071\tWebster\tND\tRamsey County\tH1\n58345\t38071\tLawton\tND\tRamsey County\tH1\n58325\t38071\tChurchs ferry\tND\tRamsey County\tH1\n58380\t38071\tTolna\tND\tRamsey County\tH1\n58229\t38071\tFairdale\tND\tRamsey County\tH1\n58355\t38071\tNekoma\tND\tRamsey County\tH1\n58057\t38073\tMcleod\tND\tRansom County\tH1\n58062\t38073\tNome\tND\tRansom County\tH1\n58490\t38073\tVerona\tND\tRansom County\tH1\n58069\t38073\tStirum\tND\tRansom County\tH1\n58068\t38073\tSheldon\tND\tRansom County\tH1\n58033\t38073\tFort ransom\tND\tRansom County\tH1\n58049\t38073\tKathryn\tND\tRansom County\tH1\n58027\t38073\tEnderlin\tND\tRansom County\tH1\n58060\t38073\tMilnor\tND\tRansom County\tH1\n58052\t38073\tLeonard\tND\tRansom County\tH1\n58054\t38073\tLisbon\tND\tRansom County\tH1\n58750\t38075\tLansford\tND\tRenville County\tH1\n58740\t38075\tGlenburn\tND\tRenville County\tH1\n58718\t38075\tBerthold\tND\tRenville County\tH1\n58734\t38075\tDonnybrook\tND\tRenville County\tH1\n58787\t38075\tTolley\tND\tRenville County\tH1\n58782\t38075\tSherwood\tND\tRenville County\tH1\n58725\t38075\tCarpio\tND\tRenville County\tH1\n58761\t38075\tMohall\tND\tRenville County\tH1\n58746\t38075\tKenmare\tND\tRenville County\tH1\n58041\t38077\tHankinson\tND\tRichland County\tH1\n58047\t38077\tHorace\tND\tRichland County\tH1\n58015\t38077\tChristine\tND\tRichland County\tH1\n58057\t38077\tMcleod\tND\tRichland County\tH1\n58077\t38077\tWalcott\tND\tRichland County\tH1\n58053\t38077\tLidgerwood\tND\tRichland County\tH1\n58058\t38077\tMantador\tND\tRichland County\tH1\n58076\t38077\tWahpeton\tND\tRichland County\tH1\n58075\t38077\tWahpeton\tND\tRichland County\tH1\n58030\t38077\tFairmount\tND\tRichland County\tH1\n58060\t38077\tMilnor\tND\tRichland County\tH1\n58052\t38077\tLeonard\tND\tRichland County\tH1\n58061\t38077\tMooreton\tND\tRichland County\tH1\n58001\t38077\tAbercrombie\tND\tRichland County\tH1\n58051\t38077\tKindred\tND\tRichland County\tH1\n58018\t38077\tColfax\tND\tRichland County\tH1\n58081\t38077\tWyndmere\tND\tRichland County\tH1\n58008\t38077\tBarney\tND\tRichland County\tH1\n58367\t38079\tRolla\tND\tRolette County\tH1\n58384\t38079\tWillow city\tND\tRolette County\tH1\n58316\t38079\tBelcourt\tND\tRolette County\tH1\n58353\t38079\tMylo\tND\tRolette County\tH1\n58363\t38079\tPerth\tND\tRolette County\tH1\n58365\t38079\tRocklake\tND\tRolette County\tH1\n58317\t38079\tBisbee\tND\tRolette County\tH1\n58369\t38079\tSaint john\tND\tRolette County\tH1\n58385\t38079\tWolford\tND\tRolette County\tH1\n58366\t38079\tRolette\tND\tRolette County\tH1\n58329\t38079\tDunseith\tND\tRolette County\tH1\n58040\t38081\tGwinner\tND\tSargent County\tH1\n58067\t38081\tRutland\tND\tSargent County\tH1\n58474\t38081\tOakes\tND\tSargent County\tH1\n58043\t38081\tHavana\tND\tSargent County\tH1\n58053\t38081\tLidgerwood\tND\tSargent County\tH1\n58069\t38081\tStirum\tND\tSargent County\tH1\n58060\t38081\tMilnor\tND\tSargent County\tH1\n58017\t38081\tCogswell\tND\tSargent County\tH1\n58013\t38081\tCayuga\tND\tSargent County\tH1\n58032\t38081\tForman\tND\tSargent County\tH1\n58054\t38081\tLisbon\tND\tSargent County\tH1\n58444\t38083\tGoodrich\tND\tSheridan County\tH1\n58736\t38083\tDrake\tND\tSheridan County\tH1\n58723\t38083\tButte\tND\tSheridan County\tH1\n58559\t38083\tMercer\tND\tSheridan County\tH1\n58463\t38083\tMcclusky\tND\tSheridan County\tH1\n58430\t38083\tDenhoff\tND\tSheridan County\tH1\n58710\t38083\tAnamoose\tND\tSheridan County\tH1\n58341\t38083\tHarvey\tND\tSheridan County\tH1\n58758\t38083\tMartin\tND\tSheridan County\tH1\n58529\t38085\tCarson\tND\tSioux County\tH1\n58528\t38085\tCannon ball\tND\tSioux County\tH1\n58570\t38085\tSolen\tND\tSioux County\tH1\n58538\t38085\tFort yates\tND\tSioux County\tH1\n58568\t38085\tSelfridge\tND\tSioux County\tH1\n58643\t38087\tMarmarth\tND\tSlope County\tH1\n58647\t38087\tNew england\tND\tSlope County\tH1\n58651\t38087\tRhame\tND\tSlope County\tH1\n58653\t38087\tScranton\tND\tSlope County\tH1\n58620\t38087\tAmidon\tND\tSlope County\tH1\n58623\t38087\tBowman\tND\tSlope County\tH1\n58649\t38087\tReeder\tND\tSlope County\tH1\n58601\t38089\tDickinson\tND\tStark County\tH1\n58638\t38089\tHebron\tND\tStark County\tH1\n58656\t38089\tTaylor\tND\tStark County\tH1\n58647\t38089\tNew england\tND\tStark County\tH1\n58655\t38089\tSouth heart\t
